vi "Read Input Registers from Slave.vi"(7 "Unit ID":u8, 8 "error in (no error)":errorcluster, 9 "length":u16, 10 "start":u16, 11 "Modbus Master in":refnum<class "Modbus Master.lvclass">) -> (0 "error out":errorcluster, 3 "register values":u16[](array[numeric]))   [LabVIEW 2021, in "Modbus Master Engine.lvlib"]
uses:
  Modbus Master Engine.lvlib
  Modbus API.lvlibp/API/Master/Modbus Master.lvclass
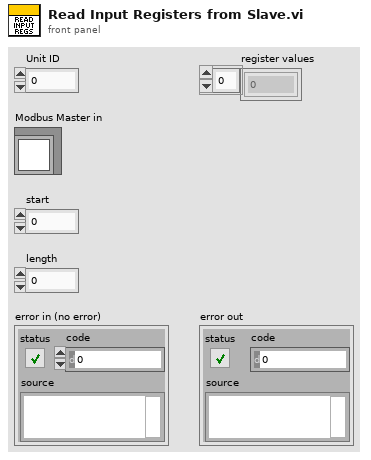
[diagram p1: front panel]
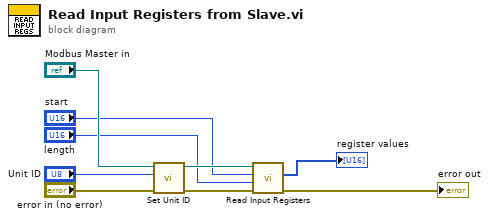
[diagram p0: block diagram]
diagram:
  n1 = call "Set Unit ID.vi"("error in"="error in (no error)", "unit ID"="Unit ID", "Modbus master in"="Modbus Master in") -> ("error out"=w8:errorcluster, "Modbus master out"=w7:refnum<class "Modbus Master.lvclass">)  [unwired: 7 in]
  n2 = call-dynamic "Read Input Registers.vi"("error in"=w8, "number of inputs"="length", "starting address"="start", "Modbus master in"=w7) -> ("error out"=→"error out":errorcluster, "register values"=→"register values":u16[])  [unwired: 5 in, 1 out]
